vi "Sixtypes Insert.vi"() -> ()   [LabVIEW 2012]
doc: "This VI shows how you can insert data of different data types into a table named sixtypes in the LabVIEW.mdb database. \n\nThe table is deleted if it already exists. A new table is created using the column names and data types defined by the column information array on the panel. The values shown at the bottom of the panel are the ones actually inserted into the table fields.\n\nYou can use the Sixtypes Select VI to read the values back from the table."
uses:
  Connection.llb/DB Tools Open Connec (Path).vi
  NI_Database_API_64.lvlib
  Auxilliary.llb/DB Tools Format Datetime String (Time Stamp).vi
  Auxilliary.llb/DB Tools DataTypes.ctl
  Auxilliary.llb/DB Tools Column Info.ctl
panel:
  out "Date/Time \n(in sec - 0 is now)":string
  in  "Binary (CDB)":cdb=12.5-98.04i format="%.2f"
  in  "Numeric (Double)":dbl=1202.556 format="%.7f"
  in  "Numeric (Single)":sgl=-0.02168 format="%.5f"
  in  "Numeric (Long)":i32=125
  in  "String":string="this is a test."
  in  "column information":T1[](array[typedef])=[{"column name"="Str", "data type"=enum."String", "size"=30, "allow null?"=FALSE}, {"column name"="I32", "data type"=enum."Long (I32)", "size"=0, "allow null?"=FALSE}, {"column name"="SGL", "data type"=enum."Single (SGL)", "size"=0, "allow null?"=FALSE}, {"column name"="DBL", "data type"=enum."Double (DBL)", "size"=0, "allow null?"=FALSE}, {"column name"="DT", "data type"=enum."Date/Time", "size"=0, "allow null?"=FALSE}, {"column name"="Bin", "data type"=enum."Binary", "size"=0, "allow null?"=FALSE}]
  # "Values"
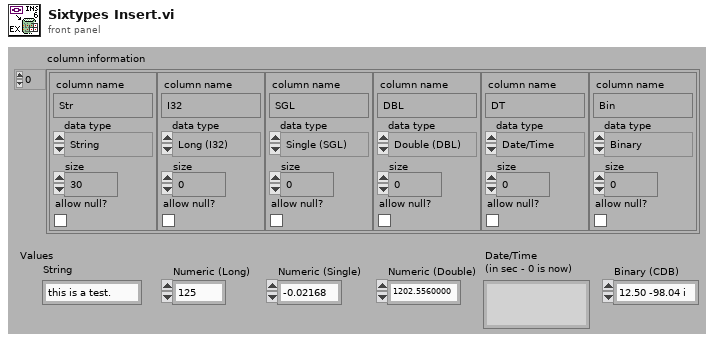
[diagram p1: front panel]
types:
  T1 = typedef "NI_Database_API_64.lvlib/DB Tools Column Info.ctl" = cluster{"column name":string, "data type":T2, "size":i32, "allow null?":bool}
  T2 = typedef "NI_Database_API_64.lvlib/DB Tools DataTypes.ctl" = enum16{"String", "Long (I32)", "Single (SGL)", "Double (DBL)", "Date/Time", "Binary"}
  T3 = typedef "NI_Database_API_64.lvlib/Conn ObjectReference.ctl" = refnum<k1>
  T4 = cluster{"String":string, "Numeric (Long)":i32, "Numeric (Single)":sgl, "Numeric (Double)":dbl, "date/time string":string, "Binary (CDB)":cdb}
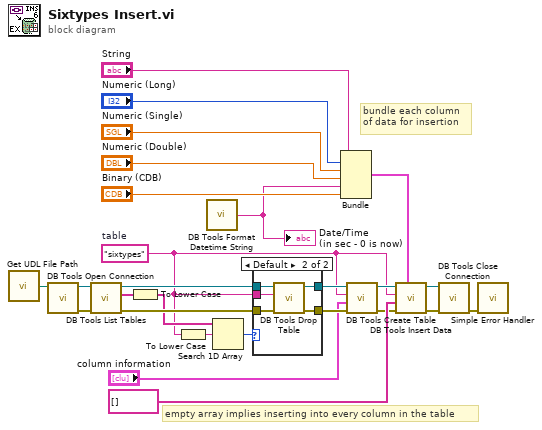
[diagram p0: block diagram]
diagram:
  w4 = "sixtypes"  # table
  # "bundle each column\nof data for insertion"
  # "empty array implies inserting into every column in the table"
  n1 = call "Get UDL File Path.vi"() -> ("UDL file path"=w2:path)  [unwired: 1 in]
  n2 = call-poly "DB Tools Open Connection.vi"("connection information"=w2) -> ("error out"=w26:errorcluster, "connection reference"=w25:T3)  [unwired: 7 in]
  n3 = call "DB Tools List Tables.vi"("error in (no error)"=w26, "connection reference"=w25) -> ("error out"=w23:errorcluster, "tables"=w24:string[], "connection reference out"=w22:T3)  [unwired: 3 in]
  n4 = To Lower Case(string=w24) -> (all lower case string=w21:string[])
  n5 = To Lower Case(string=w4) -> (all lower case string=w20:string)
  n6 = call-poly "DB Tools Format Datetime String.vi"() -> ("date/time string"=w1:string)  [unwired: 1 in]
  "Date/Time \n(in sec - 0 is now)" <- w1
  n7 = Search 1D Array(1D array=w21, element=w20) -> (index of element=w19:i32)  [unwired: 1 in]
  n8 = case shown="Default" w19 {
    tunnel: w23 -> [w27 w33]
    tunnel: w22 -> [w28 w32]
    tunnel: [w28 w31] -> w8
    tunnel: [w27 w30] -> w9
    tunnel: w4 -> [_ w29]
    frame -1 {
    }
    frame Default {
      n9 = call "DB Tools Drop Table.vi"("error in (no error)"=w33, "table"=w29, "connection reference"=w32) -> ("error out"=w30:errorcluster, "connection reference out"=w31:T3)  [unwired: 5 in]
    }
  }
  n10 = Bundle("String"="String", "Numeric (Long)"="Numeric (Long)", "Numeric (Single)"="Numeric (Single)", "Numeric (Double)"="Numeric (Double)", "date/time string"=w1, "Binary (CDB)"="Binary (CDB)") -> (w10:T4)  [unwired: 1 in]
  n11 = call "DB Tools Create Table.vi"("error in (no error)"=w9, "column information"="column information", "table"=w4, "connection reference"=w8) -> ("error out"=w6:errorcluster, "connection reference out"=w7:T3)  [unwired: 4 in]
  n12 = call "DB Tools Insert Data.vi"("data"=w10, "error in (no error)"=w6, "columns"=string[] [], "table"=w4, "connection reference"=w7) -> ("error out"=w17:errorcluster, "connection reference out"=w16:T3)  [unwired: 5 in]
  n13 = call "DB Tools Close Connection.vi"("error in (no error)"=w17, "connection reference"=w16) -> ("error out"=w3:errorcluster)  [unwired: 5 in]
  n14 = call <vilib>:"Simple Error Handler.vi"("error in (no error)"=w3) -> ()  [unwired: 4 in, 5 out]
